vi "LoginDialogUI.vi"() -> (1 "PWord":string, 2 "Cancelled":bool, 3 "UserName":string)   [LabVIEW 2022 SP3, in "Login_Dialog.lvlib" / "Login_Dialog.lvclass"]
uses:
  Login_Dialog.lvclass
panel:
  in  "Password":string caption="String"
  in  "User":string caption="String"
  in  "Cancel":bool caption="Blank"
  in  "OK":bool caption="Blank"
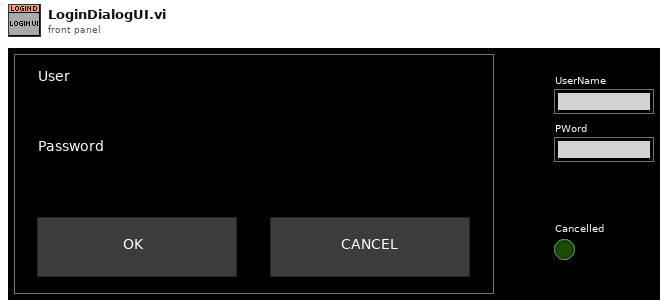
[diagram p1: front panel]
types:
  T1 = enum8{"Enabled", "Disabled", "Disabled and Grayed Out"}
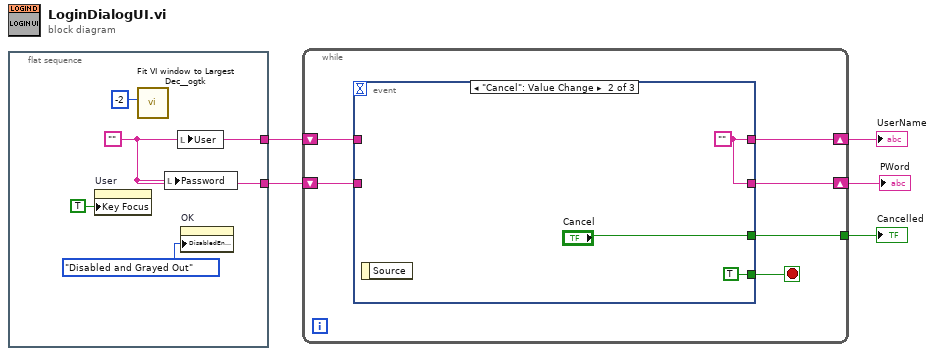
[diagram p0: block diagram]
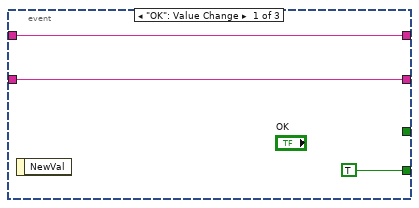
[diagram p2: hidden frame]
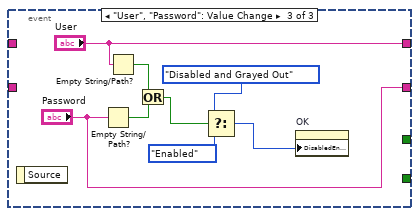
[diagram p3: hidden frame]
diagram:
  n1 = flat-sequence {
    tunnel: [w6] -> w4
    tunnel: [w6] -> w2
    frame #0 {
      w6 = ""
      n2 = property on="User" class="Str"("Key Focus"=TRUE) -> ()  [unwired: 2 in, 2 out]
      n3 = call <userlib>:"Fit VI window to Largest Dec__ogtk.vi"("border spacing (2 px)"=-2) -> ()  [unwired: 5 in, 2 out]
      n4 = local write "Password"(w6) -> ()
      n5 = local write "User"(w6) -> ()
      n6 = property on="OK" class="Bool"("DisabledEnum"=T1."Disabled and Grayed Out" ("Disabled")) -> ()  [unwired: 2 in, 2 out]
    }
  }
  n7 = while {
    tunnel: [w14] -> w5
    shift-right: [w12] -> w3
    shift-left: w4 -> [w13]
    shift-right: [w10] -> w1
    shift-left: w2 -> [w11]
    stop <- w15 stop-if-true
    n8 = event shown="[1] \"Cancel\": Value Change" {
      selector: _ -> [_ _ _]
      dyn-events: _ -> [_ _ _]
      timeout: _ -> [_ _ _]
      tunnel: [TRUE ("OK") TRUE ("OK") _] -> w15
      tunnel: [_ "Cancel" _] -> w14
      tunnel: w13 -> [w16 _ _]
      tunnel: [w16 w20 "User"] -> w12
      tunnel: [w17 w20 "Password"] -> w10
      tunnel: w11 -> [w17 _ _]
      event "OK": Value Change {
        n9 = event-data() -> ()  [unwired: 1 in, 1 out]
      }
      event "Cancel": Value Change {
        w20 = ""
        n10 = event-data() -> ()  [unwired: 1 in, 1 out]
      }
      event "User", "Password": Value Change {
        n11 = event-data() -> ()  [unwired: 1 in, 1 out]
        n12 = Empty String/Path?(string/path="Password") -> (empty?=w25:bool)
        n13 = Empty String/Path?(string/path="User") -> (empty?=w24:bool)
        n14 = Or(x=w24, y=w25) -> (x .or. y?=w23:bool)
        n15 = Select(t=T1."Disabled and Grayed Out" ("Disabled"), s=w23, f=T1."Enabled" ("Disabled")) -> (s? t:f=w27:T1)
        n16 = property on="OK" class="Bool"("DisabledEnum"=w27) -> ()  [unwired: 2 in, 2 out]
      }
    }
  }
  "Cancelled" <- w5
  "UserName" <- w3
  "PWord" <- w1
